vi "Bearing Time-Cepstrum Analysis.vi"() -> ()   [LabVIEW 2023]
doc: "This example demonstrates how to compute the time-cepstrum of a univariate time series by using the TSA Time-Cepstrum VI.\n\nIf the cepstrum of a time series changes over time, you cannot identify the periodic components and echoes of that time series by observing traditional cepstrums. In this situation, you can estimate the time-cepstrum to identify the changing cepstrum along the time axis. \n\nIn this example, the TSA Time-Cepstrum VI estimates the time-cepstrum of four types of bearing vibration signals. For both normal and abnormal bearing signals, you cannot observe cepstrum peaks in traditional cepstrums. By estimating the time-cepstrum of the normal bearing signals, the time-cepstrum does not contain obvious peaks. For abnormal bearing signals, you can observe obvious peak lines in the time-cepstrum.\n\n<b>Instructions:</b>\nRun this VI. Observe the Cepstrogram of different bearing vibration signals."
uses:
  <vilib>/Waveform/WDTOps.llb/WDT Get Final Time Value DBL.vi
  <vilib>/addons/Time Series Analysis/Correlation and Spectral Analysis.llb/TSA Time-Cepstrum (Waveform).vi
  <vilib>/addons/Time Series Analysis/Utilities.llb/TSA Configure Cepstrogram Indicator (Predefined Color Table).vi
  <vilib>/addons/_Advanced Signal Processing/NI_AdvSigProcTSA.lvlib
panel:
  in  "Bearing Signal":u16(ring) items=["Normal (nonstationary)", "Abnormal (nonstationary)", "Normal (stationary)", "Abnormal (stationary)"]
  out "Cepstrogram":dbl[][](graph)
  out "Original Signal":waveform(sgl)(graph)
  # "Overview: Demonstrates how to compute the time-cepstrum of a univariate time series by using the TSA Time-Cepstrum VI.\nRequirements: LabVIEW Full Development System, Advanced Signal Processing Toolkit\nInstructions: \nRun this VI. Observe the Cepstrogram of different bearing vibration signals."
  # "Signal Choice"
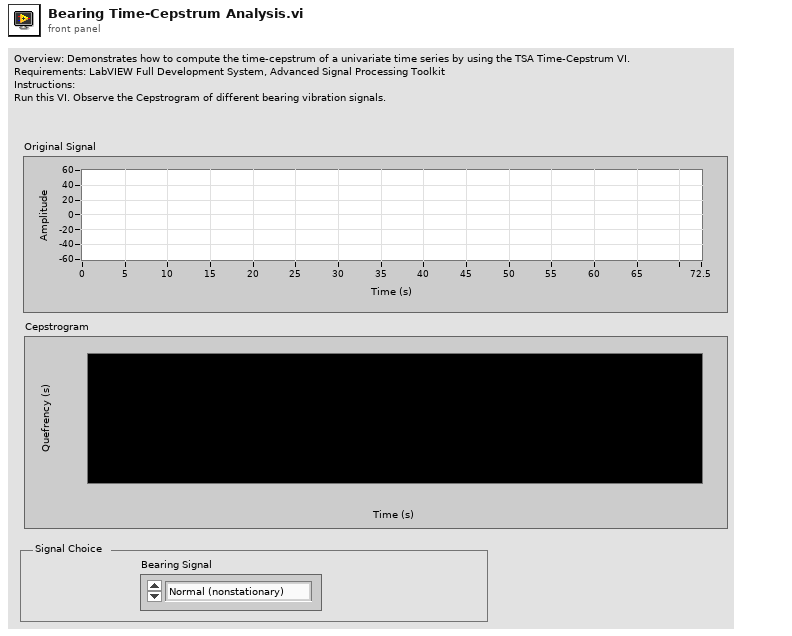
[diagram p1: front panel]
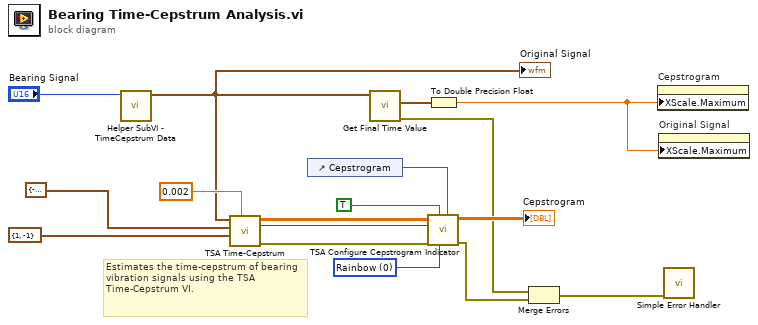
[diagram p0: block diagram]
diagram:
  w5 = u16 0 items=["Rainbow", "Inverse gray", "Gray"] ("color table")
  # "Estimates the time-cepstrum of bearing vibration signals using the TSA Time-Cepstrum VI."
  n1 = call "Helper SubVI - TimeCepstrum Data.vi"("Bearing Signal"="Bearing Signal") -> ("signal"=w4:waveform(sgl))  [unwired: 10 in]
  "Original Signal" <- w4
  n2 = call-poly <vilib>:"TSA Time-Cepstrum.vi"("quefrency offset"=0.002, "window info"=cluster{"type":i32, "length":i32} {"type"=1, "length"=-1}, "time-quefrency sampling info"=cluster{"time steps":i32, "frequency bins":i32} {"time steps"=-1, "frequency bins"=512} ("time-freq sampling info"), "Xt"=w4) -> ("error out"=w9:errorcluster, "scale info"=w6:variant, "cepstrogram"=w10:dbl[][])  [unwired: 3 in, 2 out]
  n3 = control-ref of="Cepstrogram"() -> (w13:refnum<vi>)
  n4 = call-poly <vilib>:"Get Final Time Value.vi"("waveform in"=w4) -> ("error out"=w2:errorcluster, "tf"=w8:timestamp)  [unwired: 1 in, 8 out]
  n5 = call-poly <vilib>:"TSA Configure Cepstrogram Indicator.vi"("reference of cepstrogram indicator"=w13, "color table"=w5, "dB on? (F)"=TRUE ("dB? (F)"), "error in (no error)"=w9, "scale info"=w6, "cepstrogram"=w10) -> ("error out"=w1:errorcluster, "cepstrogram indicator"=→"Cepstrogram":dbl[][])  [unwired: 1 in, 3 out]
  n6 = To Double Precision Float(number=w8) -> (double precision float=w17:dbl)
  n7 = Merge Errors(w2, w1) -> (w16:errorcluster)
  n8 = property on="Cepstrogram" class="IntGraph (strict)"("XScale.Maximum"=w17) -> ()  [unwired: 2 in, 2 out]
  n9 = property on="Original Signal" class="WFGraph (strict)"("XScale.Maximum"=w17) -> ()  [unwired: 2 in, 2 out]
  n10 = call <vilib>:"Simple Error Handler.vi"("error in (no error)"=w16) -> ()  [unwired: 4 in, 5 out]
